vi "Auto Centerize.vi"(3 "angle to horizon Y":u16=85, 4 "Camera Y ServoDeviceRef":T1={"DeviceStatus"={"status"=FALSE, "code"=0, "source"=""}, "Digital Module"=enum."Digital Module 1", "PWM Channel"=enum."Invalid", "DeadBand"={"Name"="", "maxPositivePwm"=0, "minPositivePwm"=0, "centerPwm"=0, "maxNegativePwm"=0, "minNegativePwm"=0, "angularRange"=0}}, 5 "angle to horizon X":u16=85, 6 "Camera X ServoDeviceRef":T1={"DeviceStatus"={"status"=FALSE, "code"=0, "source"=""}, "Digital Module"=enum."Digital Module 1", "PWM Channel"=enum."Invalid", "DeadBand"={"Name"="", "maxPositivePwm"=0, "minPositivePwm"=0, "centerPwm"=0, "maxNegativePwm"=0, "minNegativePwm"=0, "angularRange"=0}}) -> (0 "zAvit":dbl, 1 "X Drive Arcade":dbl, 2 "Centerized?":bool)   [LabVIEW 2012]
uses:
  <vilib>/Rock Robotics/WPI/PWM/Servo/WPI_ServoDeviceRef.ctl
  <vilib>/Rock Robotics/SystemInterfaces/Typedef/FPGA_TypedefDigitalModule.ctl
  <vilib>/Rock Robotics/SystemInterfaces/DIO/FPGA_DIOPWMChannel.ctl
  <vilib>/Rock Robotics/WPI/PWM/WPI_PWMDeadband.ctl
  BotStatus.vi
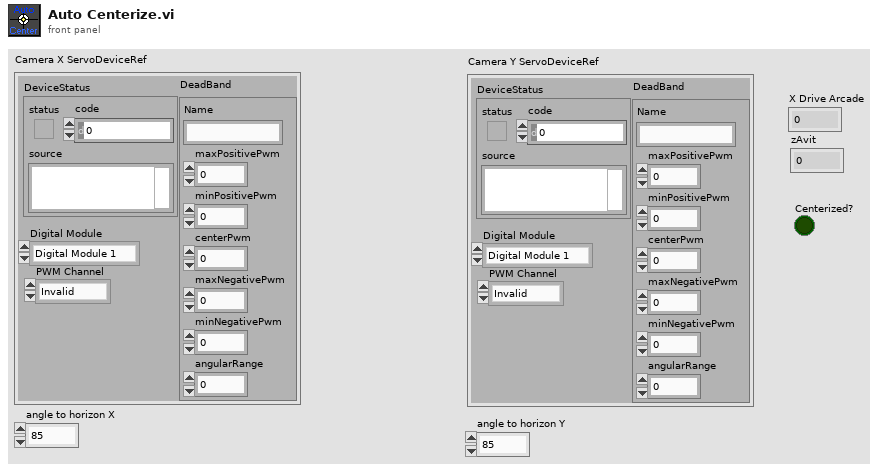
[diagram p1: front panel]
types:
  T1 = typedef "WPI_ServoDeviceRef.ctl" = cluster{"DeviceStatus":errorcluster, "Digital Module":T2, "PWM Channel":T3, "DeadBand":T4}
  T2 = typedef "FPGA_TypedefDigitalModule.ctl" = enum16{"Digital Module 1", "Digital Module 2"}
  T3 = typedef "FPGA_DIOPWMChannel.ctl" = enum8{"PWM 1", "PWM 2", "PWM 3", "PWM 4", "PWM 5", "PWM 6", "PWM 7", "PWM 8", "PWM 9", "PWM 10", "Invalid"}
  T4 = typedef "WPI_PWMDeadband.ctl" = cluster{"Name":string, "maxPositivePwm":i32, "minPositivePwm":i32, "centerPwm":i32, "maxNegativePwm":i32, "minNegativePwm":i32, "angularRange":u16}
  T5 = cluster{"Target Position X":dbl, "Target Position Y":dbl, "Target Found":bool}
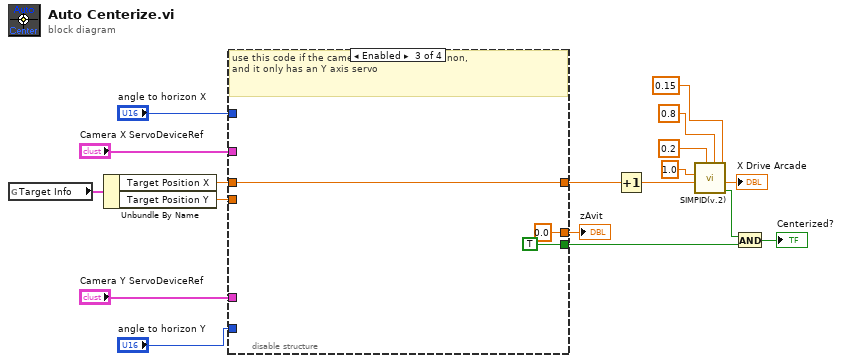
[diagram p0: block diagram]
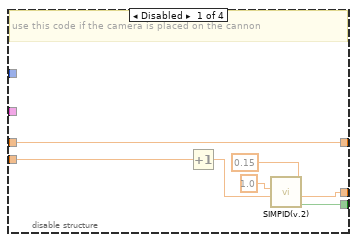
[diagram p2: hidden frame]
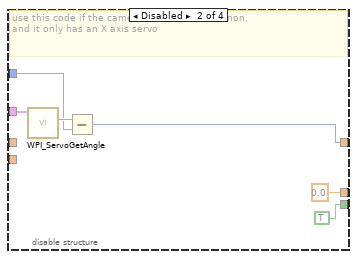
[diagram p3: hidden frame]
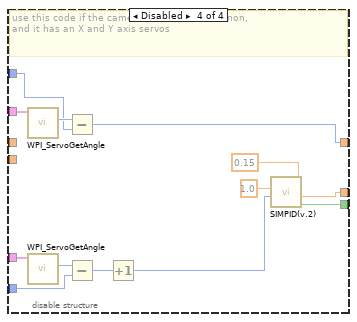
[diagram p4: hidden frame]
diagram:
  n1 = global read "BotStatus.vi" "Target Info"() -> (w16:T5)
  n2 = Unbundle By Name(w16) -> ("Target Position X"=w5:dbl, "Target Position Y"=w15:dbl)
  n3 = disable-structure shown="Enabled" {
    disable-tunnel: [w25 0.0 ("zAvit") 0.0 ("zAvit") w36] -> w18
    disable-tunnel: w15 -> [w24 _ _ _]
    disable-tunnel: [w23 TRUE ("On Target") TRUE ("On Target") w35] -> w11
    disable-tunnel: [w19 w29 w34 w41] -> w6
    disable-tunnel: w5 -> [w19 _ w34 _]
    disable-tunnel: "Camera X ServoDeviceRef" -> [_ w27 _ w46]
    disable-tunnel: "Camera Y ServoDeviceRef" -> [_ _ _ w44]
    disable-tunnel: "angle to horizon X" -> [_ w26 _ w43]
    disable-tunnel: "angle to horizon Y" -> [_ _ _ w42]
    frame Disabled {
      # "use this code if the camera is placed on the cannon"
      n4 = Increment(x=w24) -> (x+1=w22:dbl)
      n5 = call "SIMPID(v.2).vi"("Range"=0.15, "Current Point"=w22, "Set Point"=1.0) -> ("On Target"=w23:bool, "result"=w25:dbl)  [unwired: 7 in]
    }
    frame Disabled {
      # "use this code if the camera is not on the cannon,\nand it only has an X axis servo"
      n6 = call <vilib>:"WPI_ServoGetAngle.vi"("ServoDeviceRef"=w27) -> ("Angle"=w30:u16)  [unwired: 7 in, 2 out]
      n7 = Subtract(x=w30, y=w26) -> (x-y=w29:u16)
    }
    frame Enabled {
      # "use this code if the camera is not on the cannon,\nand it only has an Y axis servo"
    }
    frame Disabled {
      # "use this code if the camera is not on the cannon,\nand it has an X and Y axis servos"
      n8 = call <vilib>:"WPI_ServoGetAngle.vi"("ServoDeviceRef"=w46) -> ("Angle"=w47:u16)  [unwired: 7 in, 2 out]
      n9 = call <vilib>:"WPI_ServoGetAngle.vi"("ServoDeviceRef"=w44) -> ("Angle"=w45:u16)  [unwired: 7 in, 2 out]
      n10 = Subtract(x=w47, y=w43) -> (x-y=w41:u16)
      n11 = Subtract(x=w45, y=w42) -> (x-y=w37:u16)
      n12 = Increment(x=w37) -> (x+1=w40:u16)
      n13 = call "SIMPID(v.2).vi"("Range"=0.15, "Current Point"=w40, "Set Point"=1.0) -> ("On Target"=w35:bool, "result"=w36:dbl)  [unwired: 7 in]
    }
  }
  "zAvit" <- w18
  n14 = Increment(x=w6) -> (x+1=w13:dbl)
  n15 = call "SIMPID(v.2).vi"("Range"=0.15, "upper limit"=0.8, "lower limit"=0.2, "Current Point"=w13, "Set Point"=1.0) -> ("On Target"=w10:bool, "result"=→"X Drive Arcade":dbl)  [unwired: 5 in]
  n16 = And(x=w10, y=w11) -> (x .and. y?=→"Centerized?":bool)
